vi "Prompt for Step.vi"(8 "error in (no error)":errorcluster, 10 "Subpanel Ref":refnum<vi>, 11 "String Assertion in":refnum<class "String Assertion.lvclass">) -> (0 "error out":errorcluster, 3 "String Assertion out":refnum<class "String Assertion.lvclass">)   [LabVIEW 2020, in "MacroAssert.lvlib" / "String Assertion.lvclass"]
doc: "Displays its own window into <B>Subpanel Ref</B> for the user to enter a macro step."
uses:
  String Assertion.lvclass
  String Assertion Type.ctl
  String Comparator.ctl
  Assertion Step/Assertion Step.lvclass
panel:
  in  "Stop on Fail?":bool
  in  "Comparison Value":string
  in  "Comparison Type":T1
  out "Subtype Description":string
  in  "Object Name":string
  in  "Step Subtype":T2
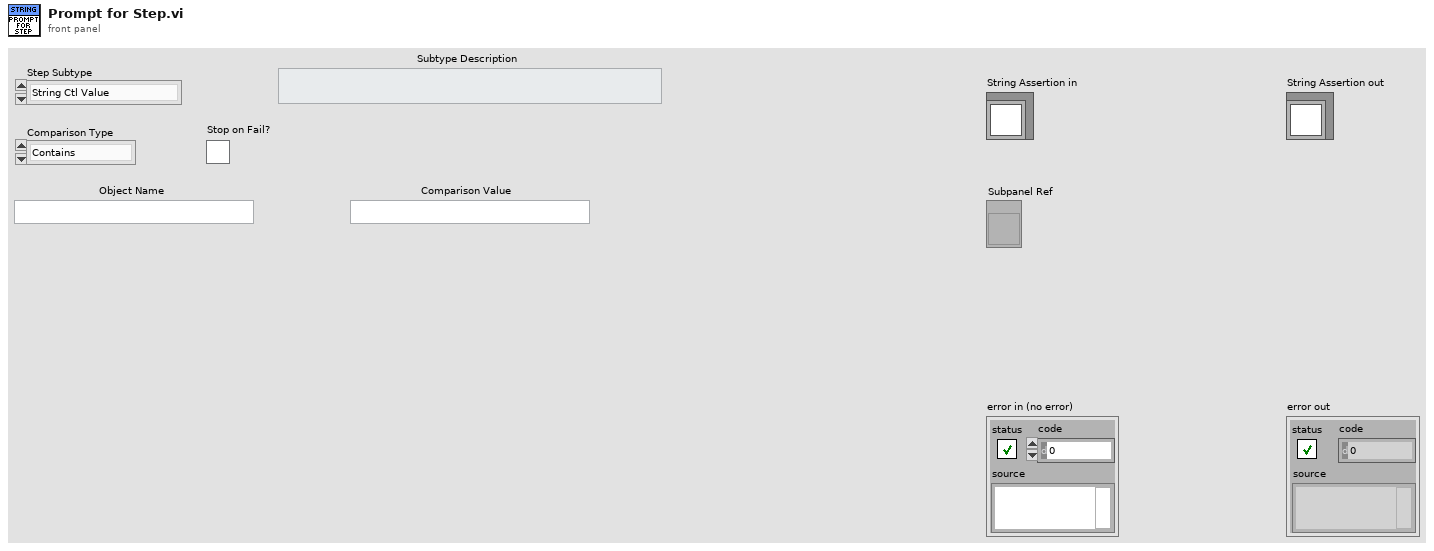
[diagram p1: front panel]
types:
  T1 = typedef "MacroAssert.lvlib/String Assertion.lvclass/String Comparator.ctl" = enum16{"Contains", "Equals", "Starts with", "Ends with", "Does not contain", "Does not equal"}
  T2 = typedef "MacroAssert.lvlib/String Assertion.lvclass/String Assertion Type.ctl" = enum16{"String Ctl Value", "Ctl Caption Property", "Ctl Tip Strip Property", "Frontmost VI Name", "Frontmost Window Name"}
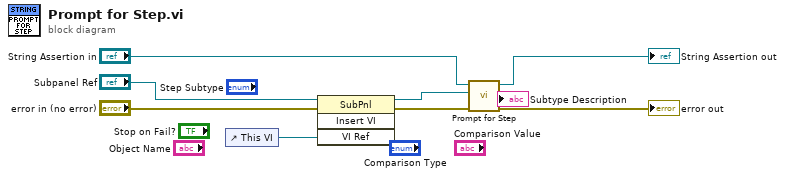
[diagram p0: block diagram]
diagram:
  n1 = control-ref of="This VI"() -> (w6:refnum<vi>)
  n2 = invoke class="SubPnl" method="Insert VI"(reference="Subpanel Ref", error in="error in (no error)", "VI Ref"=w6) -> (reference out=w7:refnum<vi>, error out=w8:errorcluster)  [unwired: 1 in, 2 out]
  n3 = call-parent "Prompt for Step.vi"("error in (no error)"=w8, "Subpanel Ref"=w7, "Step in"="String Assertion in") -> ("error out"=→"error out":errorcluster, "Step out"=→"String Assertion out":refnum<class "String Assertion.lvclass">)  [unwired: 7 in]
